vi "count_rate_group.vi"() -> ()   [LabVIEW 2017]
panel:
  out "diff array":u64[][](array[numeric])
  in  "Array":u64[](array[numeric])=[0, 1, 2, 3]
  in  "file (use dialog)":path=path "G:/tdc/2017/test_20231022_102522.dat"
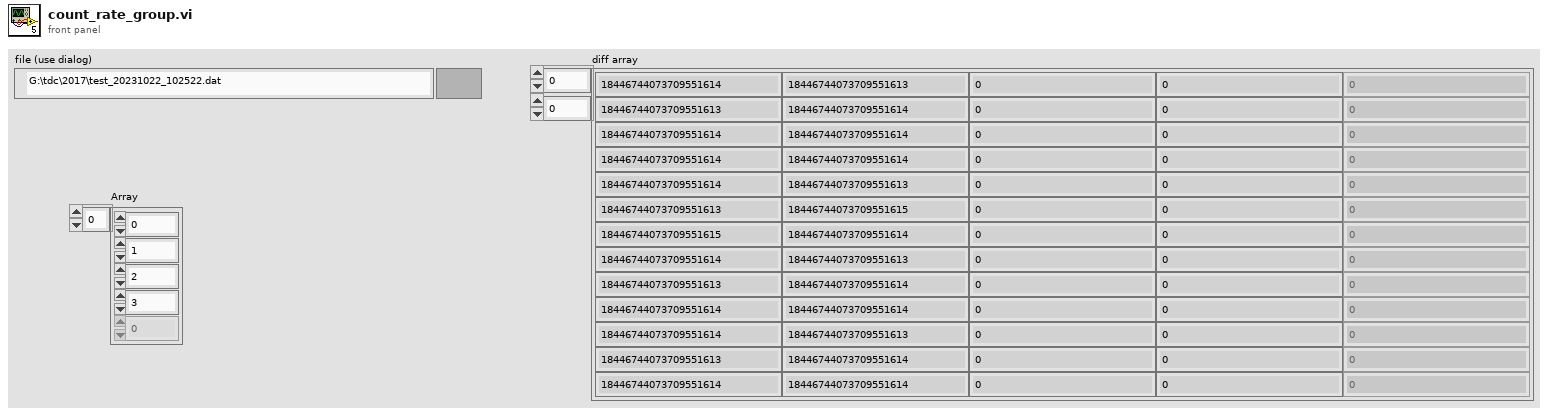
[diagram p1: front panel]
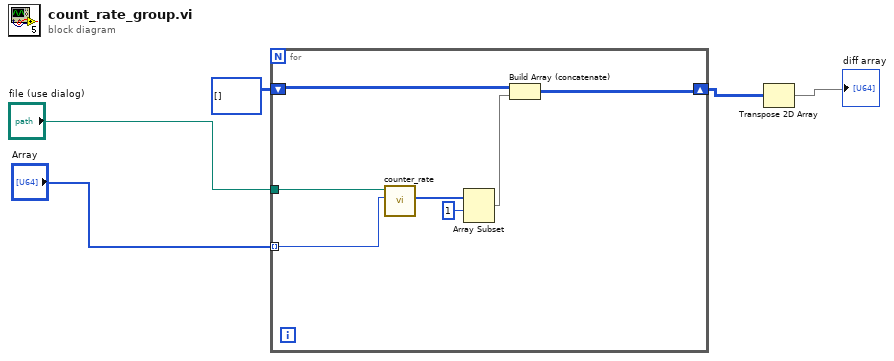
[diagram p0: block diagram]
diagram:
  n1 = for {
    tunnel: "file (use dialog)" -> [w12]
    tunnel: "Array" -> [w11] mode=indexing
    shift-right: [w9] -> w2
    shift-left: u64[][] [] -> [w10]
    n2 = call "counter_rate.vi"("channel"=w11, "file (use dialog)"=w12) -> ("diff"=w8:u64[])  [unwired: 6 in, 3 out]
    n3 = Array Subset(array=w8, index=1) -> (w6:u64[])  [unwired: 1 in]
    n4 = Build Array (concatenate)(w10, w6) -> (w9:u64[][])
  }
  n5 = Transpose 2D Array(2D array=w2) -> (transposed array=→"diff array":u64[][])
